vi "AnalogTriggerCfg.vi"(8 "error in (no error)":errorcluster, 10 "Trigger Config":T1={"Channel"=enum."chn B", "Edge"=0, "Level[V]"=0.5} {"Edge" items=["RISING", "FALLING", "ANY"]}, 11 "reference in":refnum<k24>) -> (0 "error out":errorcluster, 3 "reference out":refnum<k24>)   [LabVIEW 2019, in "LabNation Scope Driver.lvlib"]
doc: "Sets the Trigger level and Edge direction."
uses:
  LabNation Scope Driver.lvlib
  Typedef/TriggerData.ctl
  Typedef/Channel Selection.ctl
  Typedef/Edge.ctl
  C:/Program Files (x86)/LabNation/SmartScope/DeviceInterface.dll
  Program Files (x86)/LabNation/SmartScope/DeviceInterface.dll
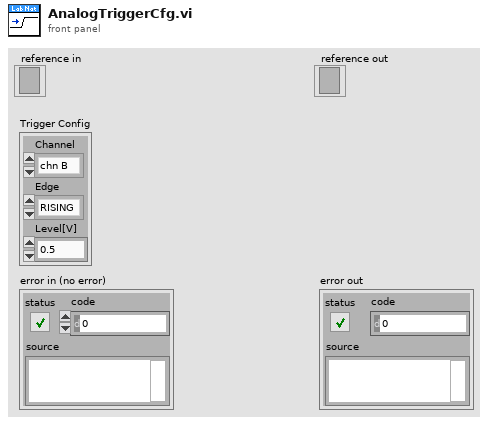
[diagram p1: front panel]
types:
  T1 = typedef "LabNation Scope Driver.lvlib/TriggerData.ctl" = cluster{"Channel":T2, "Edge":T3, "Level[V]":sgl}
  T2 = typedef "LabNation Scope Driver.lvlib/Channel Selection.ctl" = enum16{"chn A", "chn B"}
  T3 = typedef "LabNation Scope Driver.lvlib/Edge.ctl" = i32
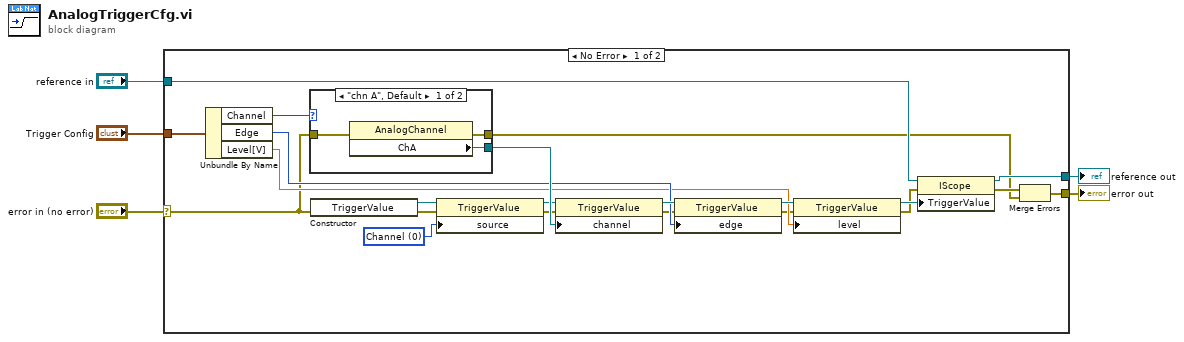
[diagram p0: block diagram]
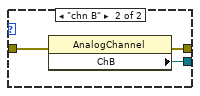
[diagram p2: hidden frame]
diagram:
  n1 = case shown="No Error" "error in (no error)" {
    selector: "error in (no error)" -> [w6 w34]
    tunnel: "reference in" -> [w20 w35]
    tunnel: [w19 w35] -> w4
    tunnel: "Trigger Config" -> [w17 _]
    tunnel: [w8 w34] -> w2
    frame No Error {
      w24 = 0 items=["Channel", "External"] ("source")
      n2 = Unbundle By Name(w17) -> ("Channel"=w16:T2, "Edge"=w15:T3, "Level[V]"=w14:sgl)
      n3 = case shown="\"chn A\", Default" w16 {
        tunnel: [w30 w33] -> w27
        tunnel: w6 -> [w28 w32]
        tunnel: [w29 w31] -> w7
        frame "chn A", Default {
          n4 = property class="AnalogChannel"(error in=w28) -> (error out=w29:errorcluster, "ChA"=w30:refnum<k24>)  [unwired: 1 in, 1 out]
        }
        frame "chn B" {
          n5 = property class="AnalogChannel"(error in=w32) -> (error out=w31:errorcluster, "ChB"=w33:refnum<k24>)  [unwired: 1 in, 1 out]
        }
      }
      n6 = constructor class="TriggerValue"(error in=w6) -> (reference out=w25:refnum<k24>, error out=w13:errorcluster)  [unwired: 2 in, 1 out]
      n7 = property class="TriggerValue"(reference=w25, error in=w13, "source"=w24) -> (reference out=w23:refnum<k24>, error out=w12:errorcluster)
      n8 = property class="TriggerValue"(reference=w23, error in=w12, "channel"=w27) -> (reference out=w22:refnum<k24>, error out=w11:errorcluster)
      n9 = property class="TriggerValue"(reference=w22, error in=w11, "edge"=w15) -> (reference out=w21:refnum<k24>, error out=w10:errorcluster)
      n10 = property class="TriggerValue"(reference=w21, error in=w10, "level"=w14) -> (reference out=w26:refnum<k24>, error out=w9:errorcluster)
      n11 = property class="IScope"(reference=w20, error in=w9, "TriggerValue"=w26) -> (reference out=w19:refnum<k24>, error out=w18:errorcluster)
      n12 = Merge Errors(w18, w7) -> (w8:errorcluster)
    }
    frame Error {
    }
  }
  "reference out" <- w4
  "error out" <- w2
